vi "IMAQdx Acquisition Template (Host) -testcount.vi"() -> ()   [LabVIEW 2016]
uses:
  <vilib>/userdefined/High Color/IMAQdx.ctl
  <vilib>/FPGAPlugInAG/roboRIO/niLvFpga_Open_roboRIO.vi
  <vilib>/rvi/interface/common/dynamic/niFpgaDynamicAddResources.vi
  <vilib>/FPGAPlugInAG/Dynamic/niLvFpga_Download_Dynamic.vi
  <vilib>/FPGAPlugInAG/Dynamic/niLvFpga_Run_Dynamic.vi
  <vilib>/Utility/error.llb/Error Cluster From Error Code.vi
  <vilib>/rvi/errors/niLvFpgaAdjustHostInterfaceError.vi
  <vilib>/rvi/interface/common/niFpgaWaitOnOcc.vi
  <vilib>/vision/EDVR.llb/IMAQ ImageToEDVR 2D U32.vi
  <vilib>/FPGAPlugInAG/Dynamic/niLvFpga_Close_Dynamic.vi
  <vilib>/rvi/interface/nirviOpenFPGA/nirviOpenFPGA.xnode
  FPGA Bitfiles/ImageProcessingw_FPGATarget_ImageProcessingw_crTOG22JuF8.lvbitx
  <vilib>/rvi/interface/nirviMethod/nirviMethod.xnode
  <vilib>/rvi/interface/nirviReadWriteControl/nirviReadWriteControl.xnode
  <vilib>/rvi/interface/nirviCloseFPGA/nirviCloseFPGA.xnode
  <vilib>/vision/driver/NI_Vision_Acquisition_Software.lvlib
  <resource>/objmgr/imaqdx.rc
  <vilib>/rvi/interface/Simulation/niFpgaSimulationCallBeginRW.vi
  <vilib>/rvi/errors/niLvFpgaMergeErrorWithErrorCode.vi
  NiFpgaLv.dll
  <vilib>/FPGAPlugInAG/Dynamic/niLvFpga_ConfigureFifo_Dynamic.vi
  <vilib>/FPGAPlugInAG/Dynamic/niLvFpga_StartFifo_Dynamic.vi
  <vilib>/FPGAPlugInAG/Dynamic/niLvFpga_ReadFifo_Dynamic.vi
  <vilib>/FPGAPlugInAG/Dynamic/niLvFpga_WriteFifo_Dynamic.vi
panel:
  out "Array out":u32[][](array[numeric])
  out "Boolean":bool=TRUE
  out "Error Out 2":errorcluster
  in  "Stop":bool
  in  "Maximum Pixels per Write":u32=261244
  out "dePixelCount":u32
  out "AllPixelCount":u32
  in  "Camera":T1="cam0"
  # "Overview: Demonstrates how to acquire an image from a camera using the IMAQdx API, transfer the image to a FPGA target for processing, and retrieve the processed image for display or further processing on the host.\nRequirements:\n- LabVIEW FPGA\n- Vision Acquisition Software\n- Vision Development Module\nInstructions:\n1. Select a Camera\n2. Run the VI."
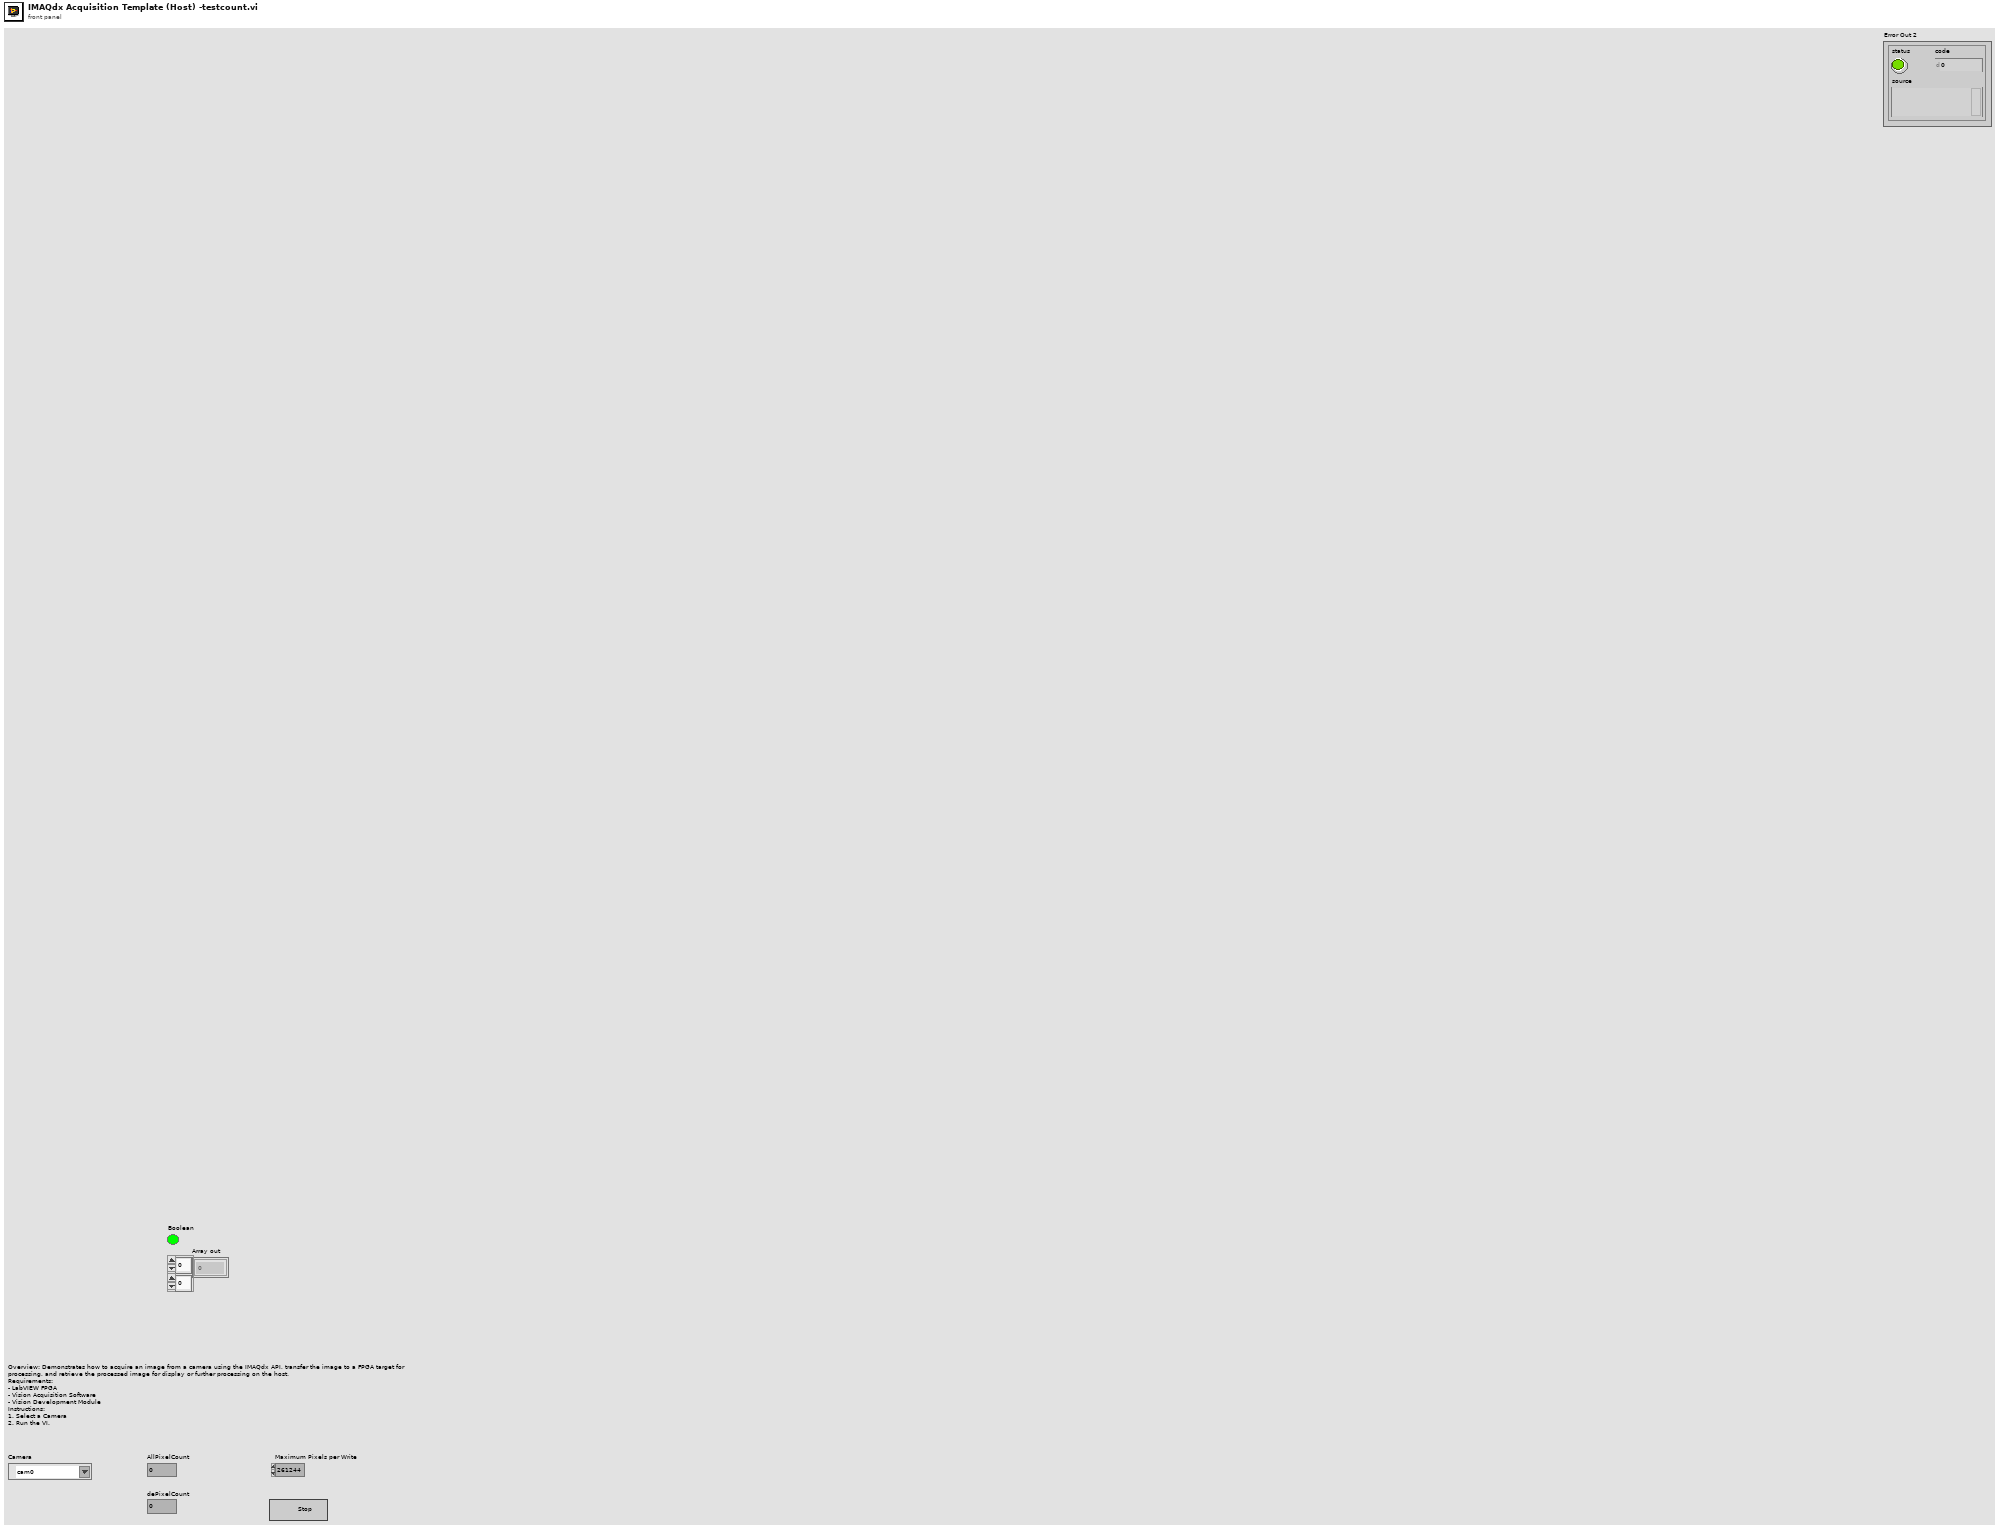
[diagram p1: front panel]
types:
  T1 = typedef "IMAQdx.ctl" = refnum<k21>
  T2 = typedef "Image Type" = u32
  T3 = typedef "IMAQ Image.ctl" = refnum<image>
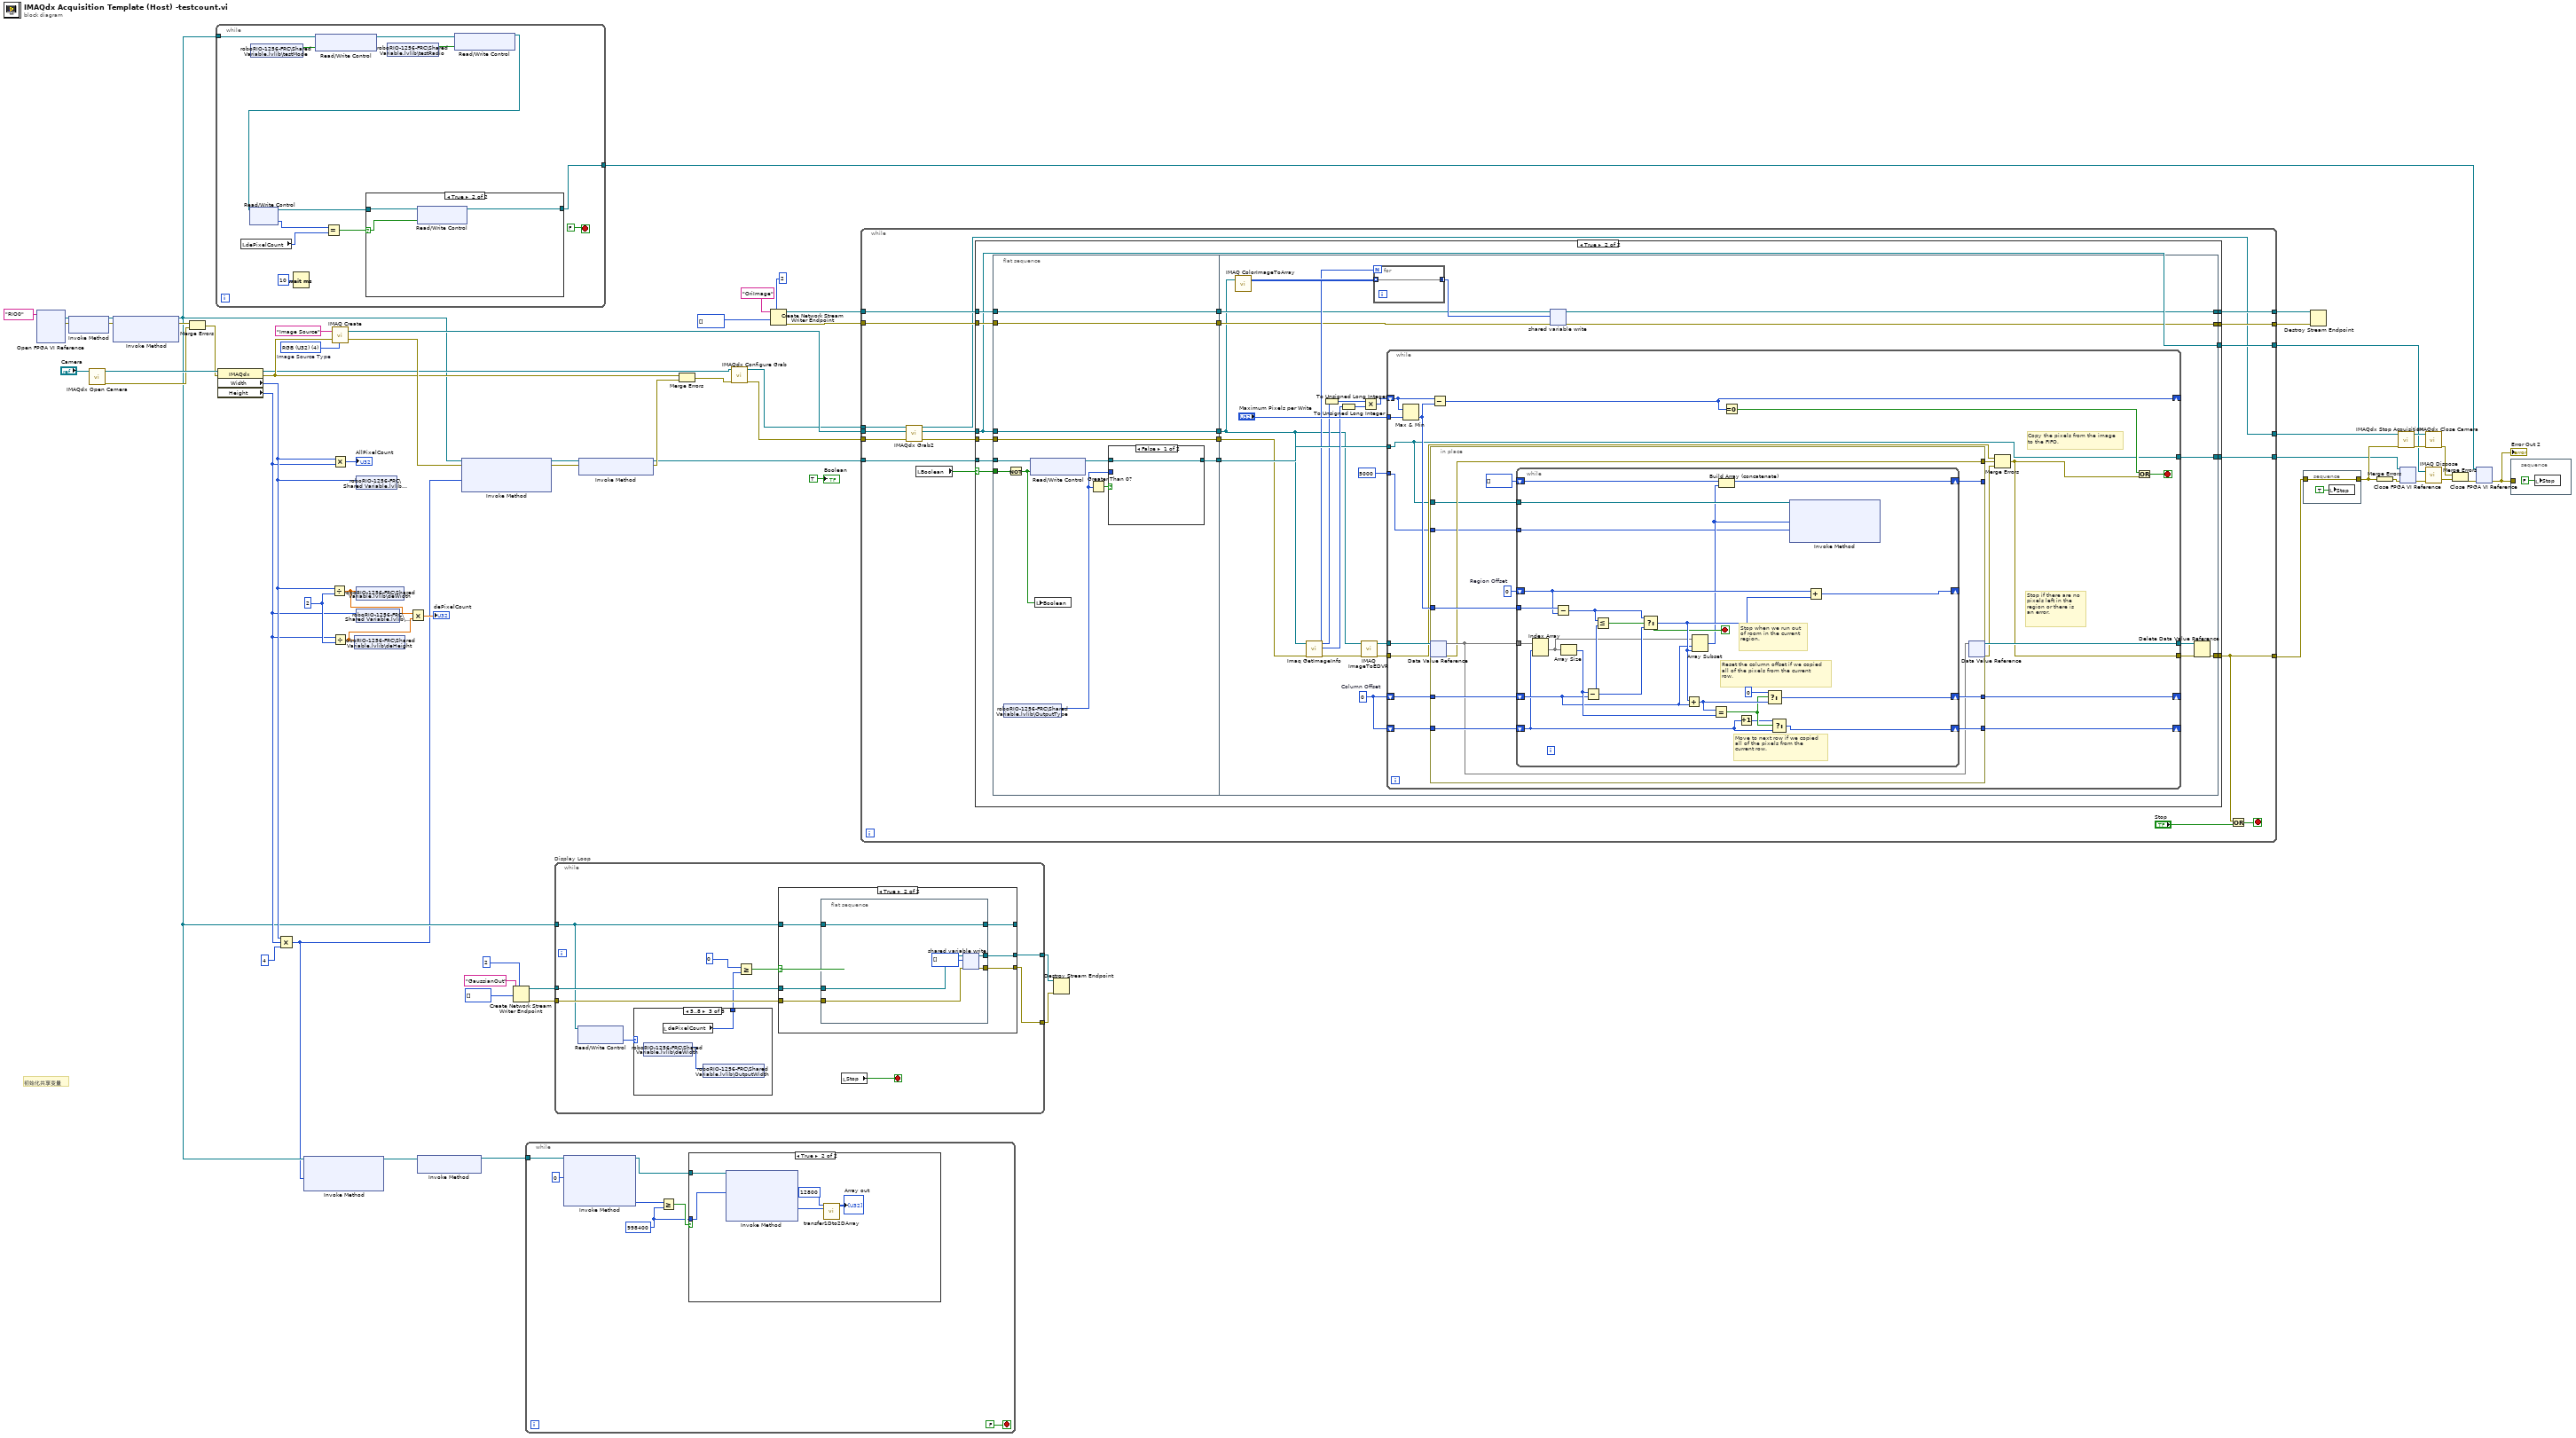
[diagram p0: block diagram]
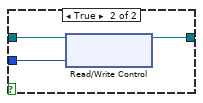
[diagram p4: hidden frame]
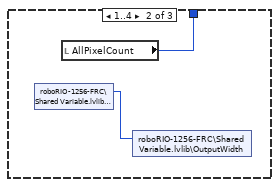
[diagram p7: hidden frame]
diagram:
  w44 = u32 2 ("y")
  w53 = T2 4 items=["Grayscale (U8)", "Grayscale (I16)", "Grayscale (SGL)", "Complex (CSG)", "RGB (U32)", "HSL (U32)", "RGB (U64)", "Grayscale (U16)"]  # Image Source Type
  # "初始化共享变量"
  n1 = xnode "Open FPGA VI Reference"("resource name"=tag "RIO0") -> ("FPGA VI Reference Out"=w60:refnum<k20>, "error out"=w61:errorcluster)  [unwired: 1 in]
  n2 = xnode "Invoke Method"("FPGA VI Reference In"=w60, "error in"=w61) -> ("FPGA VI Reference Out"=w63:refnum<k20>, "error out"=w62:errorcluster)
  n3 = call <vilib>:"IMAQdx Open Camera.vi"("Session In"="Camera") -> ("error out"=w55:errorcluster, "Session Out"=w56:T1)  [unwired: 9 in]
  n4 = xnode "Invoke Method"("FPGA VI Reference In"=w63, "error in"=w62) -> ("FPGA VI Reference Out"=w4:refnum<k20>, "error out"=w57:errorcluster)  [unwired: 1 in]
  n5 = Merge Errors(w57, w55) -> (w54:errorcluster)
  n6 = while {
    tunnel: w4 -> [w74]
    tunnel: [w70] -> w12
    stop <- FALSE stop-if-true
    n7 = local read "dePixelCount"() -> (w65:u32)
    n8 = shared-variable "roboRIO-1256-FRC\\Shared Variable.lvlib\\testMode"() -> (w73:bool)  [unwired: 1 in, 1 out]
    n9 = Wait (ms)(milliseconds to wait=u32 10) -> ()  [unwired: 1 out]
    n10 = xnode "Read/Write Control"("FPGA VI Reference In"=w74, "Mode LED Status"=w73) -> ("FPGA VI Reference Out"=w72:refnum<k20>)  [unwired: 1 in, 1 out]
    n11 = shared-variable "roboRIO-1256-FRC\\Shared Variable.lvlib\\testRadio"() -> (w71:bool)  [unwired: 1 in, 1 out]
    n12 = xnode "Read/Write Control"("FPGA VI Reference In"=w72, "Radio LED Status"=w71) -> ("FPGA VI Reference Out"=w68:refnum<k20>)  [unwired: 1 in, 1 out]
    n13 = xnode "Read/Write Control"("FPGA VI Reference In"=w68) -> ("FPGA VI Reference Out"=w67:refnum<k20>, "Count"=w66:u32)  [unwired: 1 in, 1 out]
    n14 = Equal?(x=w66, y=w65) -> (x = y?=w69:bool)
    n15 = case shown="True" w69 {
      selector: w69 -> [_ w78]
      tunnel: w67 -> [w77 w80]
      tunnel: [w77 w79] -> w70
      frame False {
      }
      frame True {
        n16 = xnode "Read/Write Control"("FPGA VI Reference In"=w80, "StartOfImage"=w78) -> ("FPGA VI Reference Out"=w79:refnum<k20>)  [unwired: 1 in, 1 out]
      }
    }
  }
  n17 = property class="IMAQdx"(reference=w56, error in=w54) -> (reference out=w9:T1, error out=w34:errorcluster, "Width"=w43:u32, "Height"=w42:u32)
  n18 = Compound Arithmetic op=MULTIPLY(w43, w42, u32 4 ("value")) -> (w3:u32)
  n19 = xnode "Invoke Method"("FPGA VI Reference In"=w4, "Requested Depth"=w3) -> ("FPGA VI Reference Out"=w2:refnum<k20>)  [unwired: 1 in, 2 out]
  n20 = Divide(x=w43, y=w44) -> (x/y=w39:dbl)
  n21 = call "IMAQ Create"("Image Name"="Image Source", "Image Type"=w53, "error in (no error)"=w34) -> ("New Image"=w10:T3, "error out"=w37:errorcluster)  [unwired: 2 in]
  n22 = Multiply(x=w43, y=w42) -> (x*y=→"AllPixelCount":u32)
  n23 = Divide(x=w42, y=w44) -> (x/y=w38:dbl)
  n24 = shared-variable "roboRIO-1256-FRC\\Shared Variable.lvlib\\deHeight"(w38) -> ()  [unwired: 1 in, 1 out]
  n25 = shared-variable "roboRIO-1256-FRC\\Shared Variable.lvlib\\Width"(w43) -> ()  [unwired: 1 in, 1 out]
  n26 = shared-variable "roboRIO-1256-FRC\\Shared Variable.lvlib\\deWidth"(w39) -> ()  [unwired: 1 in, 1 out]
  n27 = shared-variable "roboRIO-1256-FRC\\Shared Variable.lvlib\\Height"(w42) -> ()  [unwired: 1 in, 1 out]
  n28 = Multiply(x=w39, y=w38) -> (x*y=→"dePixelCount":dbl)
  n29 = xnode "Invoke Method"("FPGA VI Reference In"=w2) -> ("FPGA VI Reference Out"=w1:refnum<k20>)  [unwired: 1 in, 1 out]
  n30 = xnode "Invoke Method"("FPGA VI Reference In"=w4, "error in"=w37, "Requested Depth"=w3) -> ("FPGA VI Reference Out"=w36:refnum<k20>, "error out"=w35:errorcluster)  [unwired: 1 out]
  n31 = Create Network Stream Writer Endpoint(7:2 ("writer buffer size"), 9:i32[] [], 11:"GaussianOut" ("writer name")) -> (0:w48:errorcluster, 3:w47:refnum<k21>)  [unwired: 4 in]
  n32 = while {
    tunnel: w1 -> [w87]
    stop <- FALSE stop-if-true
    w82 = u32 998400 ("y")
    n33 = xnode "Invoke Method"("FPGA VI Reference In"=w87, "Number of Elements"=u32 0) -> ("FPGA VI Reference Out"=w83:refnum<k20>, "Elements Remaining"=w85:u32)  [unwired: 2 in, 2 out]
    n34 = Greater Or Equal?(x=w85, y=w82) -> (x >= y?=w84:bool)
    n35 = case shown="True" w84 {
      tunnel: w83 -> [_ w92]
      tunnel: w82 -> [_ w91]
      frame False {
      }
      frame True {
        n36 = xnode "Invoke Method"("FPGA VI Reference In"=w92, "Number of Elements"=w91) -> ("Data"=w90:u64[])  [unwired: 2 in, 3 out]
        n37 = call "transfer1Dto2DArray.vi"("Array in"=w90, "Width"=u16 12800) -> ("Array out"=→"Array out":i32[][])  [unwired: 9 in]
      }
    }
  }
  n38 = while "Display Loop" {
    tunnel: w4 -> [w96]
    tunnel: [w98] -> w50
    tunnel: [w101] -> w49
    tunnel: w48 -> [w100]
    tunnel: w47 -> [w99]
    stop <- w102 stop-if-true
    n39 = xnode "Read/Write Control"("FPGA VI Reference In"=w96) -> ("OutputType"=w95:u8)  [unwired: 1 in, 2 out]
    n40 = case shown="5..8" w95 {
      tunnel: [_ w104 w106] -> w94
      frame 0, Default {
      }
      frame 1..4 {
        n41 = shared-variable "roboRIO-1256-FRC\\Shared Variable.lvlib\\Width"() -> (w103:u16)  [unwired: 1 in, 1 out]
        n42 = local read "AllPixelCount"() -> (w104:u32)
        n43 = shared-variable "roboRIO-1256-FRC\\Shared Variable.lvlib\\OutputWidth"(w103) -> ()  [unwired: 1 in, 1 out]
      }
      frame 5..8 {
        n44 = shared-variable "roboRIO-1256-FRC\\Shared Variable.lvlib\\deWidth"() -> (w105:u16)  [unwired: 1 in, 1 out]
        n45 = local read "dePixelCount"() -> (w106:u32)
        n46 = shared-variable "roboRIO-1256-FRC\\Shared Variable.lvlib\\OutputWidth"(w105) -> ()  [unwired: 1 in, 1 out]
      }
    }
    n47 = Greater Or Equal?(x=u32 0, y=w94) -> (x >= y?=w97:bool)
    n48 = case shown="True" w97 {
      tunnel: w96 -> [w107 w115]
      tunnel: [w109 w114] -> w101
      tunnel: w100 -> [w108 w113]
      tunnel: w99 -> [w109 w112]
      tunnel: [w108 w111] -> w98
      tunnel: [w107 w110] -> _
      frame False {
      }
      frame True {
        n49 = flat-sequence {
          tunnel: [w120] -> w114
          tunnel: [w117] -> w111
          tunnel: [w121] -> w110
          tunnel: w115 -> [w121]
          tunnel: w113 -> [w119]
          tunnel: w112 -> [w118]
          frame #0 {
            n50 = shared-variable-write(w118, w119, i32[] [] ("data in")) -> (w120:refnum<k21>, w117:errorcluster)  [unwired: 1 in, 1 out]
          }
        }
      }
    }
    n51 = local read "Stop"() -> (w102:bool)
  }
  n52 = xnode "Invoke Method"("FPGA VI Reference In"=w36, "error in"=w35) -> ("FPGA VI Reference Out"=w11:refnum<k20>, "error out"=w33:errorcluster)
  n53 = Merge Errors(w34, w33) -> (w8:errorcluster)
  n54 = call <vilib>:"IMAQdx Configure Grab.vi"("error in"=w8, "Session In"=w9) -> ("error out"=w6:errorcluster, "Session Out"=w7:T1)  [unwired: 8 in]
  n55 = Create Network Stream Writer Endpoint(7:2 ("writer buffer size"), 9:i32[] [], 11:"OriImage" ("writer name")) -> (0:w26:errorcluster, 3:w27:refnum<k21>)  [unwired: 4 in]
  n56 = while {
    tunnel: [w136] -> w32
    tunnel: [w135] -> w31
    tunnel: w27 -> [w134]
    tunnel: w26 -> [w133]
    tunnel: [w128] -> w16
    tunnel: w7 -> [w125]
    tunnel: w10 -> [w124]
    tunnel: w6 -> [w123]
    tunnel: w11 -> [w129]
    tunnel: [w132] -> w14
    tunnel: [w131] -> w15
    tunnel: [w130] -> w13
    stop <- w137 stop-if-true
    n57 = call <vilib>:"IMAQdx Grab2.vi"("error in"=w123, "Image In"=w124, "Session In"=w125) -> ("error out"=w126:errorcluster, "Image Out"=w127:T3, "Session Out"=w128:T1)  [unwired: 5 in, 1 out]
    n58 = local read "Boolean"() -> (w122:bool)
    n59 = case shown="True" w122 {
      selector: w122 -> [_ w144]
      tunnel: w129 -> [w140 w158]
      tunnel: w127 -> [w141 w150]
      tunnel: [w139 w157] -> w132
      tunnel: [w143 w156] -> w136
      tunnel: [w142 w155] -> w135
      tunnel: w134 -> [w143 w154]
      tunnel: w133 -> [w142 w153]
      tunnel: w126 -> [w139 w152]
      tunnel: [w140 w151] -> w131
      tunnel: [w141 w150] -> w130
      frame False {
      }
      frame True {
        n60 = flat-sequence {
          tunnel: w150 -> [w166]
          tunnel: w152 -> [w167]
          tunnel: w153 -> [w168]
          tunnel: w154 -> [w169]
          tunnel: w158 -> [w164]
          tunnel: [w162] -> w149
          tunnel: [w169] -> w148
          tunnel: [w168] -> w147
          tunnel: [w167] -> w146
          tunnel: [w166] -> w145
          tunnel: w144 -> [w165]
          tunnel: [w182] -> w157
          tunnel: [w180] -> w156
          tunnel: [w179] -> w155
          tunnel: [w175] -> w151
          tunnel: w149 -> [w185]
          tunnel: w148 -> [w178]
          tunnel: w147 -> [w177]
          tunnel: w146 -> [w176]
          tunnel: w145 -> [w174]
          frame #0 {
            n61 = shared-variable "roboRIO-1256-FRC\\Shared Variable.lvlib\\OutputType"() -> (w160:u8)  [unwired: 1 in, 1 out]
            n62 = Not(x=w165) -> (.not. x?=w159:bool)
            n63 = xnode "Read/Write Control"("FPGA VI Reference In"=w164, "CanSendImage"=w159) -> ("FPGA VI Reference Out"=w163:refnum<k20>)  [unwired: 1 in, 1 out]
            n64 = local write "Boolean"(w159) -> ()
            n65 = Greater Than 0?(x=w160) -> (x > 0?=w161:bool)
            n66 = case shown="False" w161 {
              tunnel: w163 -> [w170 w173]
              tunnel: [w170 w172] -> w162
              tunnel: w160 -> [_ w171]
              frame False {
              }
              frame True {
                n67 = xnode "Read/Write Control"("FPGA VI Reference In"=w173, "OutputType"=w171) -> ("FPGA VI Reference Out"=w172:refnum<k20>)  [unwired: 1 in, 1 out]
              }
            }
          }
          frame #1 {
            w187 = u32 0  # Column Offset
            n68 = call "IMAQ ColorImageToArray"("Image"=w174) -> ("Image Pixels (U32)"=w184:u32[][])  [unwired: 3 in, 2 out]
            n69 = call "Imaq GetImageInfo"("error in (no error)"=w176, "Image"=w174) -> ("error out"=w193:errorcluster, "Y Resolution"=w194:i32, "X Resolution"=w183:i32)  [unwired: 2 in, 5 out]
            n70 = To Unsigned Long Integer(number=w183) -> (unsigned 32bit integer=w196:u32)
            n71 = To Unsigned Long Integer(number=w194) -> (unsigned 32bit integer=w197:u32)
            n72 = call-poly <vilib>:"IMAQ ImageToEDVR.vi"("error out"=w193, "Image"=w174) -> ("error out"=w191:errorcluster, "EDVR 2D U32"=w192:refnum<data-value>)  [unwired: 7 in, 1 out]
            n73 = Multiply(x=w196, y=w197) -> (x*y=w188:u32)
            n74 = for {
              N: w183 -> [_]
              tunnel: w184 -> [w198] mode=indexing
              tunnel: [w198] -> w181 mode=concatenating
            }
            n75 = while {
              shift-right: [w210] -> _
              shift-left: w188 -> [w207]
              tunnel: w192 -> [w216]
              shift-right: [w212] -> _
              shift-left: w187 -> [w214]
              shift-right: [w215] -> _
              shift-left: w187 -> [w213]
              tunnel: w185 -> [w200]
              tunnel: [w211] -> w190
              tunnel: [w202] -> w189
              tunnel: "Maximum Pixels per Write" -> [w206]
              tunnel: 5000 ("Write Timeout (ms)") -> [w199]
              tunnel: w191 -> [w201]
              tunnel: [w200] -> w175
              stop <- w209 stop-if-true
              # "Copy the pixels from the image\nto the FIFO."
              # "Stop if there are no\npixels left in the \nregion or there is\nan error."
              n76 = Max & Min(x=w207, y=w206) -> (min(x,y)=w205:u32)  [unwired: 1 out]
              n77 = in-place {
                in-place-border: w205 -> [w226]
                in-place-border: [w228] -> w215
                in-place-border: w214 -> [w225]
                in-place-border: w213 -> [w223]
                in-place-border: [w224] -> w212
                in-place-border: [w220] -> w204
                in-place-border: [w219] -> _
                in-place-border: w200 -> [w218]
                in-place-border: w199 -> [w217]
                w227 = u32 0  # Region Offset
                n78 = in-place-dvr #1(w216) -> (w222:u32[][], w220:errorcluster)
                n79 = while {
                  tunnel: w222 -> [w237]
                  shift-right: [w249] -> _
                  shift-left: w227 -> [w248]
                  tunnel: w226 -> [w251]
                  shift-right: [w242] -> w224
                  shift-left: w225 -> [w238]
                  shift-right: [w233] -> w219
                  shift-left: u8[] [] -> [w234]
                  shift-right: [w239] -> w228
                  shift-left: w223 -> [w235]
                  tunnel: w218 -> [w231]
                  tunnel: w217 -> [w229]
                  stop <- w232 stop-if-true
                  # "Stop when we run out\nof room in the current\nregion."
                  # "Reset the column offset if we copied\nall of the pixels from the current\nrow."
                  # "Move to next row if we copied\nall of the pixels from the\ncurrent row."
                  n80 = Index Array(array=w237, index (row)=w235) -> (element=w236:u32[])  [unwired: 1 in]
                  n81 = Subtract(x=w251, y=w248) -> (x-y=w250:u32)
                  n82 = Array Size(array=w236) -> (size(s)=w247:i32)
                  n83 = Subtract(x=w247, y=w238) -> (x-y=w245:u32)
                  n84 = Less Or Equal?(x=w250, y=w245) -> (x <= y?=w232:bool)
                  n85 = Select(t=w250, s=w232, f=w245) -> (s? t:f=w246:u32)
                  n86 = Add(x=w246, y=w238) -> (x+y=w243:u32)
                  n87 = Array Subset(array=w236, index=w238, length=w246) -> (w230:u32[])
                  n88 = Equal?(x=w243, y=w247) -> (x = y?=w241:bool)
                  n89 = Build Array (concatenate)(w234, w230) -> (w233:u32[])
                  n90 = Increment(x=w235) -> (x+1=w240:u32)
                  n91 = Select(t=u32 0 ("Elements In Region"), s=w241, f=w243) -> (s? t:f=w242:u32)
                  n92 = Select(t=w240, s=w241, f=w235) -> (s? t:f=w239:u32)
                  n93 = xnode "Invoke Method"("FPGA VI Reference In"=w231, "Data"=w230, "Timeout (ms)"=w229) -> ()  [unwired: 1 in, 3 out]
                  n94 = Add(x=w248, y=w246) -> (x+y=w249:u32)
                }
                n95 = in-place-dvr #1(w222) -> (w211:refnum<data-value>, w203:errorcluster)
              }
              n96 = Subtract(x=w207, y=w205) -> (x-y=w210:u32)
              n97 = Equal To 0?(x=w210) -> (x = 0?=w208:bool)
              n98 = Merge Errors(w201, w204, w203) -> (w202:errorcluster)
              n99 = Or(x=w208, y=w202) -> (x .or. y?=w209:bool)
            }
            n100 = shared-variable-write(w178, w177, w181) -> (w180:refnum<k21>, w179:errorcluster)  [unwired: 1 in, 1 out]
            n101 = Delete Data Value Reference(data value reference=w190, error in=w189) -> (error out=w182:errorcluster)  [unwired: 1 out]
          }
        }
      }
    }
    n102 = Or(x=w132, y="Stop") -> (x .or. y?=w137:bool)
  }
  n103 = Destroy Stream Endpoint(8:w50, 11:w49) -> ()  [unwired: 1 out]
  n104 = stacked-sequence {
    tunnel: w14 -> [w252]
    tunnel: [w252] -> w17
    frame #0 {
      n105 = local write "Stop"(TRUE ("Stop")) -> ()
    }
  }
  n106 = Destroy Stream Endpoint(8:w31, 11:w32) -> ()  [unwired: 1 out]
  n107 = Merge Errors(w17) -> (w18:errorcluster)
  n108 = call <vilib>:"IMAQdx Stop Acquisition.vi"("error in"=w17, "Session In"=w16) -> ("error out"=w22:errorcluster, "Session Out"=w23:T1)  [unwired: 8 in]
  n109 = xnode "Close FPGA VI Reference"("FPGA VI Reference In"=w15, "error in"=w18) -> ("error out"=w25:errorcluster)
  n110 = call <vilib>:"IMAQdx Close Camera.vi"("error in"=w22, "Session In"=w23) -> ("error out"=w21:errorcluster)  [unwired: 9 in]
  n111 = call "IMAQ Dispose"("Image"=w13, "error in (no error)"=w25) -> ("error out"=w24:errorcluster)  [unwired: 4 in]
  n112 = Merge Errors(w21, w24) -> (w20:errorcluster)
  n113 = xnode "Close FPGA VI Reference"("FPGA VI Reference In"=w12, "error in"=w20) -> ("error out"=w19:errorcluster)
  "Error Out 2" <- w19
  n114 = stacked-sequence {
    tunnel: w19 -> [_]
    frame #0 {
      n115 = local write "Stop"(FALSE ("Stop")) -> ()
    }
  }
  "Boolean" <- TRUE
